vi "ex_FileReadAll.vi"(0 "Parsing Data and Options In":T5={"chunk in"="", "file_params"={"include col headings?"=FALSE, "x_columns"=0, "col headings always?"=FALSE, "time preference"=0, "hide col headings"=FALSE}, "delimiter"="", "optional info"={"description"="", "operator"="", "project"=""}, "Generic Header In"=[], "channel info"=[], "read segment header in"=FALSE, "# of samples read (in)"=0, "# of samples to read"=0, "# of samples in Channel Group"=0, "file refs in"={"file ref"=refnum, "file size (bytes:0)"=0, "read pointer (bytes:0)"=0, "chunk size (bytes:65000)"=65000}, "origin timestamp"=timestamp(0 s since 1904-01-01), "Is generic text file"=FALSE, "Decimal Separator"=""} {"origin timestamp" format="%<%X\n%x>T"; "channel info"."Delta X" format="%.2p"; "channel info"."X0" format="%<%X\n%x>T"; "channel info"."Timestamp" format="%<%X\n%x>T"; "file_params"."time preference" items=["Absolute", "Relative"]; "file_params"."x_columns" items=["None", "One", "Multiple"]}, 1 "Generic File Read Parameters":T6={"Delimiter"=",", "First Row is Channel Names"=FALSE, "First Column is Time Channel"=FALSE, "Decimal Point"=0, "Start Row"=1}, 2 "Attempt to Read Generic Text Files":bool, 3 "first_time?":bool, 4 "file dialog?":bool, 5 "error in (no error)":errorcluster, 6 "file path in":path, 7 "use specified sample size":bool, 8 "Samples to read":i32=-1, 9 "relative time?":bool) -> (12 "optional info":T1, 13 "end-of-file?":bool, 14 "Parsing Data and Options Out":T5 {"channel info"."Delta X" format="%.2p"; "channel info"."X0" format="%<%X\n%x>T"; "channel info"."Timestamp" format="%<%X\n%x>T"; "file_params"."time preference" items=["Absolute", "Relative"]; "file_params"."x_columns" items=["None", "One", "Multiple"]}, 15 "Signals":waveform(dbl)[](array[waveform]), 16 "File Timestamp":timestamp, 17 "Description":string, 18 "Comment":string, 19 "error out":errorcluster)   [LabVIEW 2020]
uses:
  <vilib>/express/express input/ExFileReadBlock.llb/ex_ReadFileGenericParams.ctl
  <vilib>/express/express input/ExFileReadBlock.llb/ex_ReadFileParams.ctl
  <vilib>/express/express shared/ExFile.llb/ex_AllChanInfo.ctl
  <vilib>/express/express shared/ExFile.llb/ex_FileReference.ctl
panel:
  out "notes":string
  out "test info":T7
  out "UUT info":T8
  out "pck special blks":string[](array[string])
  out "special blocks":string[](array[string])
  # "Not used"
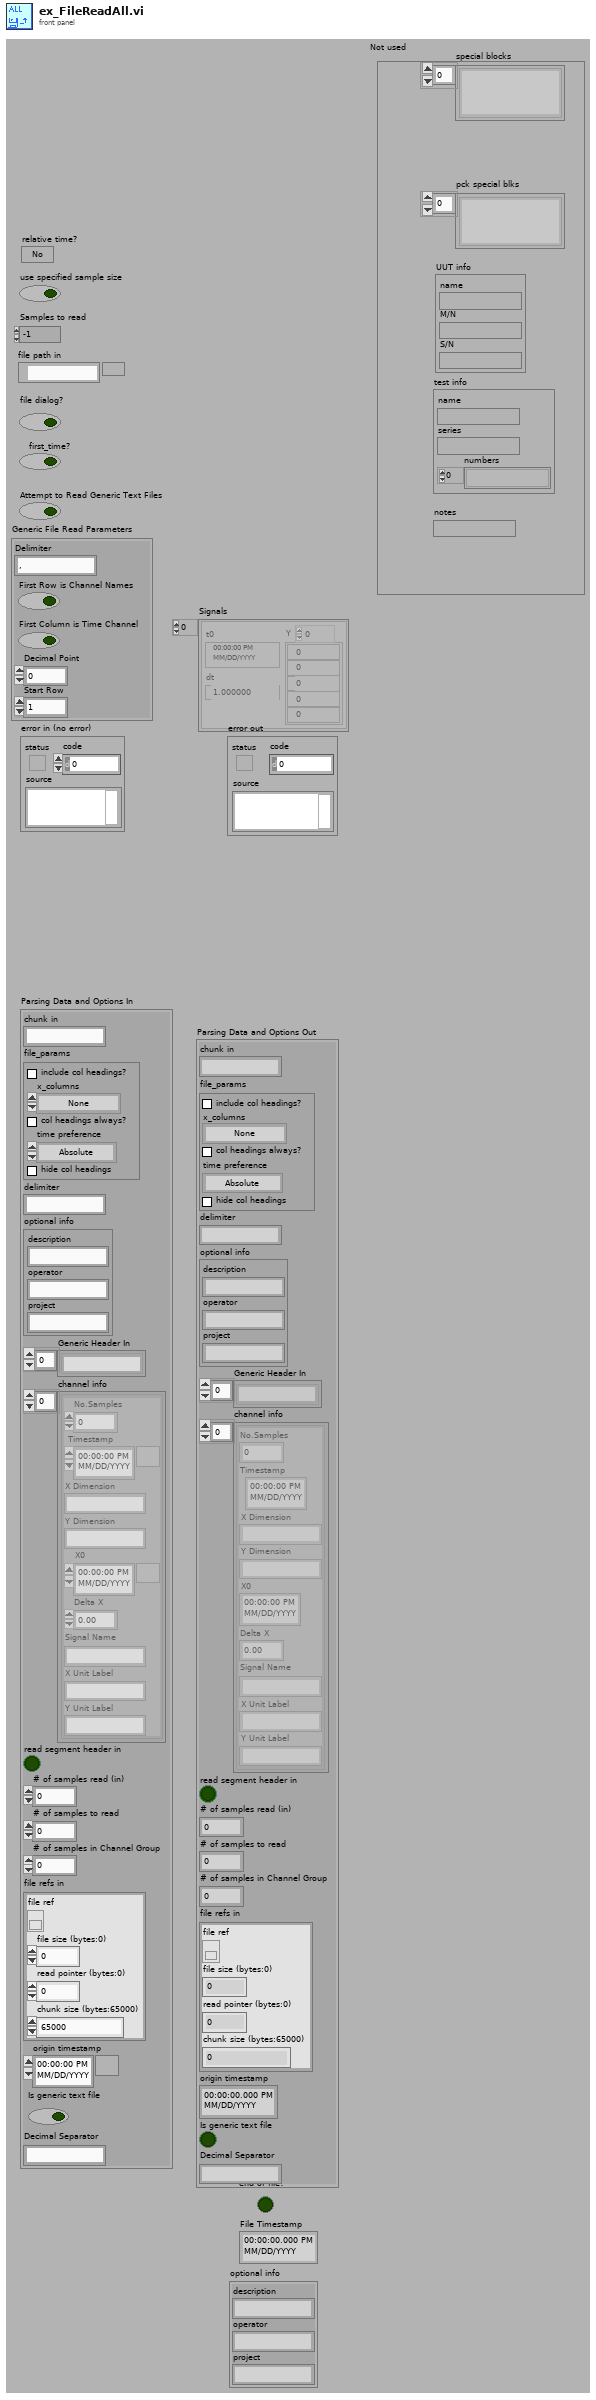
[diagram p1: front panel]
types:
  T1 = cluster{"description":string, "operator":string, "project":string}
  T2 = typedef "ex_ReadFileParams.ctl" = cluster{"include col headings?":bool, "x_columns":u16, "col headings always?":bool, "time preference":u16, "hide col headings":bool}
  T3 = typedef "ex_AllChanInfo.ctl" = cluster{"No.Samples":i32, "Timestamp":timestamp, "X Dimension":string, "Y Dimension":string, "X0":timestamp, "Delta X":dbl, "Signal Name":string, "X Unit Label":string, "Y Unit Label":string}
  T4 = typedef "ex_FileReference.ctl" = cluster{"file ref":refnum<file>, "file size (bytes:0)":i32, "read pointer (bytes:0)":i32, "chunk size (bytes:65000)":i32}
  T5 = cluster{"chunk in":string, "file_params":T2, "delimiter":string, "optional info":cluster{"description":string, "operator":string, "project":string}, "Generic Header In":string[], "channel info":T3[], "read segment header in":bool, "# of samples read (in)":u32, "# of samples to read":i32, "# of samples in Channel Group":i32, "file refs in":T4, "origin timestamp":timestamp, "Is generic text file":bool, "Decimal Separator":string}
  T6 = typedef "ex_ReadFileGenericParams.ctl" = cluster{"Delimiter":string, "First Row is Channel Names":bool, "First Column is Time Channel":bool, "Decimal Point":i32, "Start Row":i32}
  T7 = cluster{"name":string, "series":string, "numbers":string[]}
  T8 = cluster{"name":string, "M/N":string, "S/N":string}
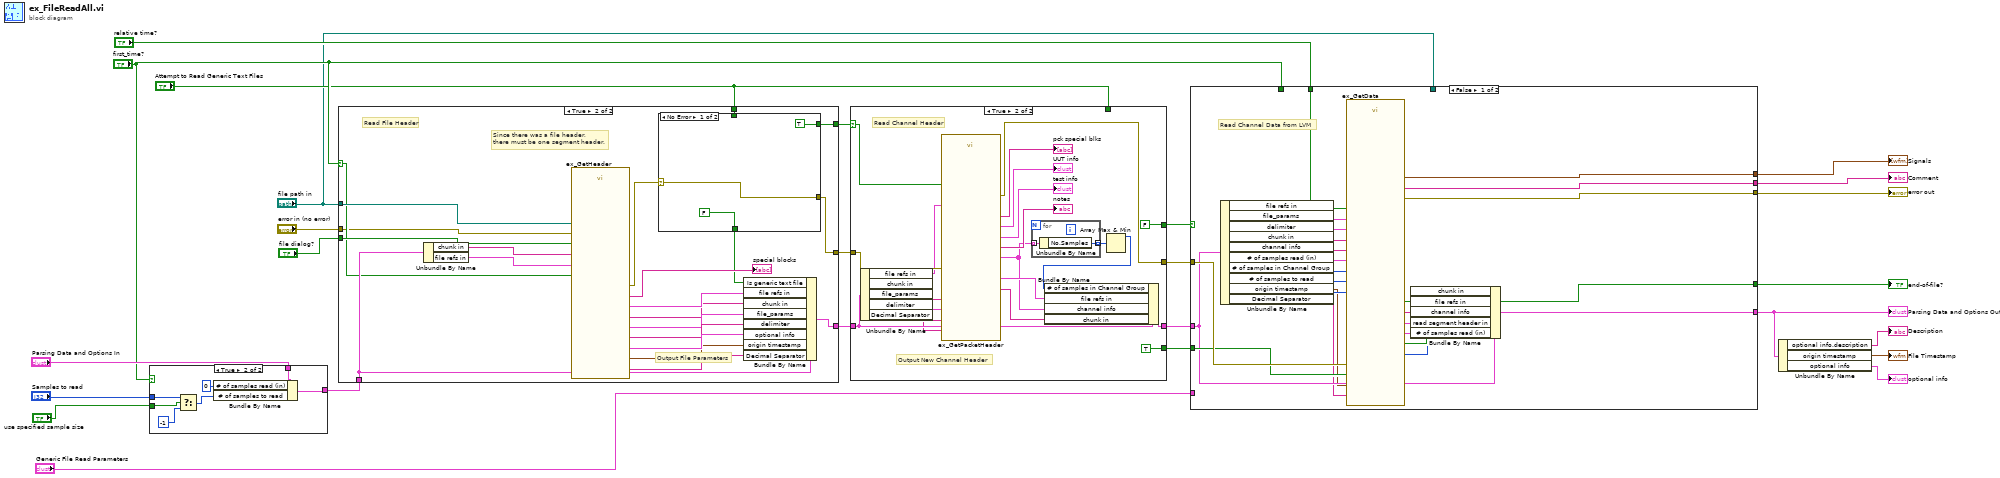
[diagram p0: block diagram]
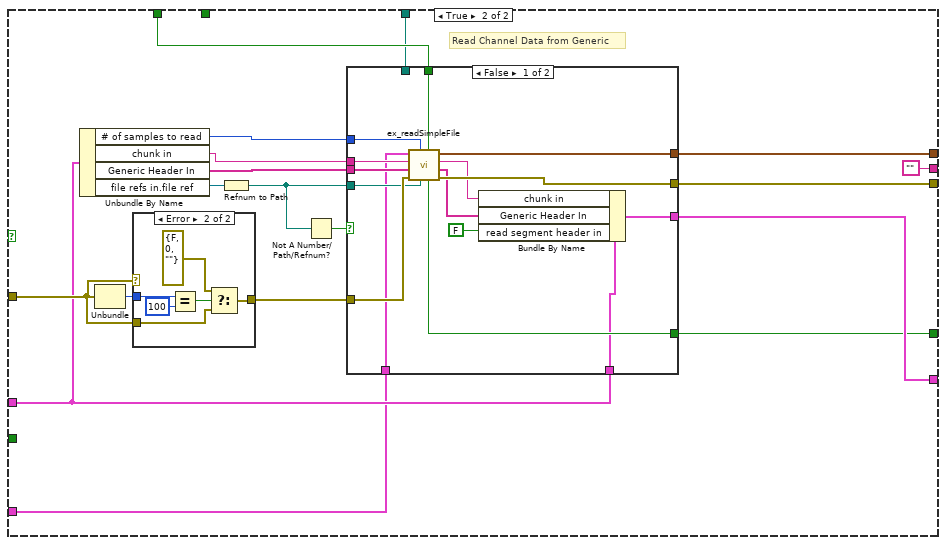
[diagram p3: hidden frame]
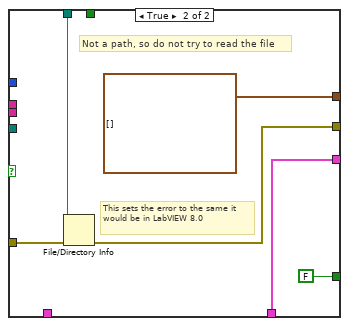
[diagram p4: hidden frame]
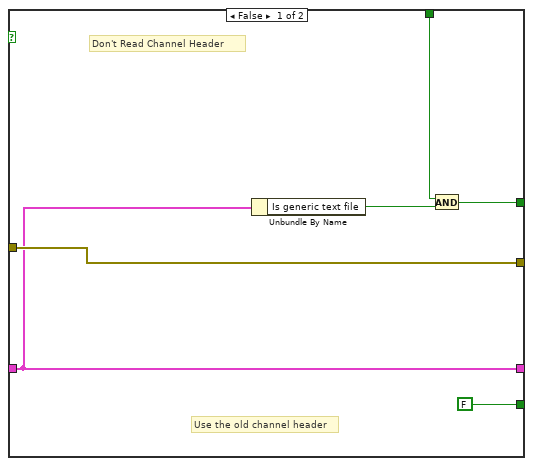
[diagram p6: hidden frame]
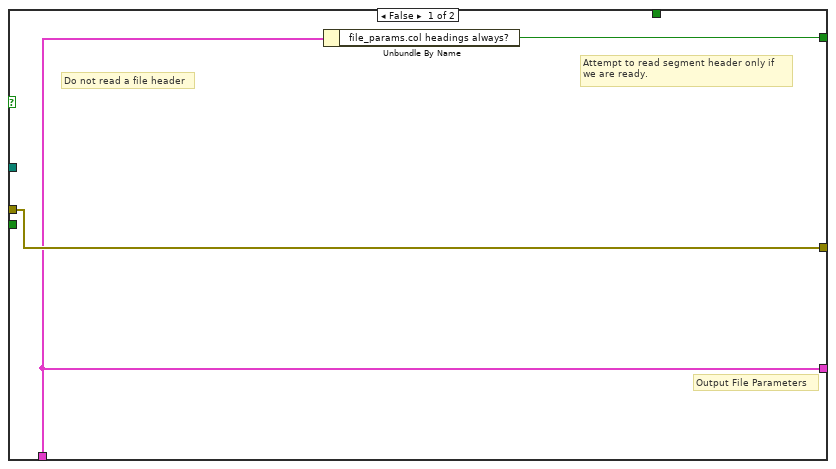
[diagram p7: hidden frame]
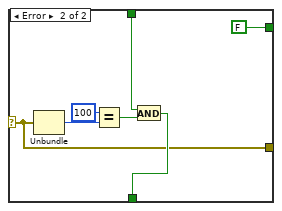
[diagram p8: hidden frame]
diagram:
  n1 = case shown="True" "first_time?" {
    tunnel: [w27 w34] -> w13
    tunnel: "Parsing Data and Options In" -> [w27 w33]
    tunnel: "Samples to read" -> [_ w29]
    tunnel: "use specified sample size" -> [_ w28]
    frame False {
    }
    frame True {
      n2 = Select(t=w29, s=w28, f=-1 ("# of samples to read")) -> (s? t:f=w30:i32)
      n3 = Bundle By Name(cluster=w33, "# of samples read (in)"=u32 0, "# of samples to read"=w30) -> (w34:T5)
    }
  }
  n4 = case shown="True" "first_time?" {
    selector: "first_time?" -> [_ w47]
    tunnel: [w35 w58] -> w14
    tunnel: "error in (no error)" -> [w37 w39]
    tunnel: [w37 w42] -> w19
    tunnel: w13 -> [w36 w49]
    tunnel: [w36 w57] -> w18
    tunnel: "file path in" -> [_ w52]
    tunnel: "file dialog?" -> [_ w51]
    tunnel: "Attempt to Read Generic Text Files" -> [_ w40]
    frame False {
      # "Attempt to read segment header only if\nwe are ready."
      # "Output File Parameters"
      # "Do not read a file header"
      n5 = Unbundle By Name(w36) -> ("file_params.col headings always?"=w35:bool)
    }
    frame True {
      # "Since there was a file header, \nthere must be one segment header."
      # "Output File Parameters"
      # "Read File Header"
      n6 = Unbundle By Name(w49) -> ("chunk in"=w50:string, "file refs in"=w48:T4)
      n7 = call <vilib>:"ex_GetHeader.vi"("file path"=w52, "file refs in"=w48, "file dialog?"=w51, "chunk in"=w50, "first_time?"=w47, "error in (no error)"=w39) -> ("Decimal Separator"=w38:string, "hdr special blks"=→"special blocks":string[], "optional info"=w55:T1, "file_params"=w53:T2, "delimiter"=w54:string, "chunk remainder"=w41:string, "file refs out"=w46:T4, "origin timestamp"=w45:timestamp, "error out"=w43:errorcluster)  [unwired: 1 out]
      n8 = case shown="No Error" w43 {
        selector: w43 -> [w59 w62]
        tunnel: [TRUE ("y") FALSE ("y")] -> w58
        tunnel: [FALSE w63] -> w44
        tunnel: [w59 w62] -> w42
        tunnel: w40 -> [_ w65]
        frame No Error {
        }
        frame Error {
          n9 = Unbundle(w62) -> ("code"=w67:i32)  [unwired: 2 out]
          n10 = Equal?(x=100, y=w67) -> (x = y?=w64:bool)
          n11 = And(x=w65, y=w64) -> (x .and. y?=w63:bool)
        }
      }
      n12 = Bundle By Name(cluster=w49, "Is generic text file"=w44, "file refs in"=w46, "chunk in"=w41, "file_params"=w53, "delimiter"=w54, "optional info"=w55, "origin timestamp"=w45, "Decimal Separator"=w38) -> (w57:T5)
    }
  }
  n13 = case shown="True" w14 {
    selector: w14 -> [_ w82]
    tunnel: w19 -> [w74 w89]
    tunnel: w18 -> [w72 w95]
    tunnel: [w72 w94] -> w16
    tunnel: [w74 w84] -> w17
    tunnel: [FALSE ("first_packet?") TRUE ("first_packet?")] -> w15
    tunnel: "Attempt to Read Generic Text Files" -> [w70 _]
    tunnel: [w69 FALSE] -> w6
    frame False {
      # "Use the old channel header"
      # "Don't Read Channel Header"
      n14 = Unbundle By Name(w72) -> ("Is generic text file"=w71:bool)
      n15 = And(x=w70, y=w71) -> (x .and. y?=w69:bool)
    }
    frame True {
      # "Output New Channel Header"
      # "Read Channel Header"
      n16 = Unbundle By Name(w95) -> ("file refs in"=w81:T4, "chunk in"=w90:string, "file_params"=w91:T2, "delimiter"=w92:string, "Decimal Separator"=w75:string)
      n17 = call <vilib>:"ex_GetPacketHeader.vi"("chunk in"=w90, "Enable"=w82, "Decimal Separator"=w75, "delimiter"=w92, "file refs in"=w81, "file_params"=w91, "error in"=w89) -> ("pck special blks"=→"pck special blks":string[], "file refs out"=w83:T4, "channel info out"=w76:T3[], "chunk remainder"=w77:string, "UUT info"=→"UUT info":T8, "test info"=→"test info":T7, "notes"=→"notes":string, "error out"=w84:errorcluster)  [unwired: 1 out]
      n18 = for {
        tunnel: w76 -> [w97] mode=indexing
        tunnel: [w96] -> w80 mode=indexing
        n19 = Unbundle By Name(w97) -> ("No.Samples"=w96:i32)
      }
      n20 = Array Max & Min(array=w80) -> (max value=w79:i32)  [unwired: 3 out]
      n21 = Bundle By Name(cluster=w95, "# of samples in Channel Group"=w79, "file refs in"=w83, "channel info"=w76, "chunk in"=w77) -> (w94:T5)
    }
  }
  n22 = case shown="False" w6 {
    tunnel: w17 -> [w111 w129]
    tunnel: w16 -> [w103 w126]
    tunnel: [w121 w137] -> w5
    tunnel: [w119 w138] -> w26
    tunnel: [w120 w139] -> w25
    tunnel: "Generic File Read Parameters" -> [_ w125]
    tunnel: "first_time?" -> [_ w136]
    tunnel: "relative time?" -> [w117 _]
    tunnel: [w118 ""] -> w21
    tunnel: [w113 w133] -> w20
    tunnel: w15 -> [w109 _]
    tunnel: "file path in" -> [_ w123]
    frame False {
      # "Read Channel Data from LVM"
      n23 = Unbundle By Name(w103) -> ("file refs in"=w116:T4, "file_params"=w115:T2, "delimiter"=w114:string, "chunk in"=w112:string, "channel info"=w100:T3[], "# of samples read (in)"=w106:u32, "# of samples in Channel Group"=w108:i32, "# of samples to read"=w107:i32, "origin timestamp"=w102:timestamp, "Decimal Separator"=w98:string)
      n24 = call <vilib>:"ex_GetData.vi"("channel info in"=w100, "chunk in"=w112, "# of samples to read (all: -1)"=w107, "file refs in"=w116, "# of samples read"=w106, "delimiter"=w114, "# of samples in channel group"=w108, "error in"=w111, "Decimal Separator"=w98, "file_params"=w115, "first_packet?"=w109, "origin timestamp"=w102, "relative time?"=w117) -> ("end-of-file?"=w113:bool, "Comment"=w118:string, "channel info out"=w99:T3[], "chunk remainder"=w101:string, "Samples read out"=w104:u32, "file refs out"=w110:T4, "Signals"=w119:waveform(dbl)[], "error out"=w120:errorcluster, "read segment header"=w105:bool)  [unwired: 6 out]
      n25 = Bundle By Name(cluster=w103, "chunk in"=w101, "file refs in"=w110, "channel info"=w99, "read segment header in"=w105, "# of samples read (in)"=w104) -> (w121:T5)
    }
    frame True {
      # "Read Channel Data from Generic"
      n26 = Unbundle By Name(w126) -> ("# of samples to read"=w132:i32, "chunk in"=w131:string, "Generic Header In"=w135:string[], "file refs in.file ref"=w127:refnum<file>)
      n27 = Unbundle(w129) -> ("code"=w130:i32)  [unwired: 2 out]
      n28 = case shown="Error" w129 {
        selector: w129 -> [w161 _]
        tunnel: w130 -> [_ w167]
        tunnel: w129 -> [_ w163]
        tunnel: [w161 w162] -> w128
        frame No Error {
        }
        frame Error {
          n29 = Equal?(x=w167, y=100) -> (x = y?=w165:bool)
          n30 = Select(t=errorcluster {"status"=FALSE, "code"=0, "source"=""} ("error out"), s=w165, f=w163) -> (s? t:f=w162:errorcluster)
        }
      }
      n31 = Refnum to Path(1:w127) -> (0:w124:path)
      n32 = Not A Number/Path/Refnum?(number/path/refnum=w124) -> (NaN/Path/Refnum?=w122:bool)
      n33 = case shown="False" w122 {
        tunnel: [w154 w157] -> w139
        tunnel: [w153 waveform(dbl)[] [] ("Signals")] -> w138
        tunnel: [w151 w159] -> w137
        tunnel: w136 -> [w150 _]
        tunnel: w135 -> [w149 _]
        tunnel: [w147 FALSE ("EOF")] -> w133
        tunnel: w132 -> [w146 _]
        tunnel: w131 -> [w145 _]
        tunnel: w128 -> [w143 w160]
        tunnel: w124 -> [w142 _]
        tunnel: w126 -> [w141 w159]
        tunnel: w125 -> [w140 _]
        tunnel: w123 -> [_ w155]
        frame False {
          n34 = call <vilib>:"ex_readSimpleFile.vi"("first time"=w150, "Path"=w142, "number of lines (all:-1)"=w146, "error in"=w143, "Generic Header In"=w149, "string in"=w145, "Generic Params"=w140) -> ("error out"=w154:errorcluster, "Generic Header Out"=w148:string[], "string remainder"=w152:string, "Signals"=w153:waveform(dbl)[], "EOF"=w147:bool)
          n35 = Bundle By Name(cluster=w141, "chunk in"=w152, "Generic Header In"=w148, "read segment header in"=FALSE) -> (w151:T5)
        }
        frame True {
          # "This sets the error to the same it would be in LabVIEW 8.0"
          # "Not a path, so do not try to read the file"
          n36 = File/Directory Info(path=w155, error in=w160) -> (error out=w157:errorcluster)  [unwired: 6 out]
        }
      }
    }
  }
  "Signals" <- w26
  "error out" <- w25
  "Comment" <- w21
  "end-of-file?" <- w20
  "Parsing Data and Options Out" <- w5
  n37 = Unbundle By Name(w5) -> ("optional info.description"=→"Description":string, "origin timestamp"=→"File Timestamp":timestamp, "optional info"=→"optional info":T1)
